vi "Self Execution.vi"(6 "Any Data":variant, 8 "error in (no error)":errorcluster, 9 "Composite Task In":refnum<class "Composite Task.lvclass">, 10 "Message In":refnum<class "Message.lvclass">, 11 "Actor In":refnum<class "System Actor.lvclass">) -> (0 "error out":errorcluster, 1 "Composite Task Out":refnum<class "Composite Task.lvclass">, 2 "Message Out":refnum<class "Message.lvclass">)   [LabVIEW 2019, in "Composite Task.lvclass"]
uses:
  Composite Task.lvclass
  Actor/System Actor/System Actor.lvclass
  Message/Message.lvclass
  Messenger/Messenger/Messenger.lvclass
  Message/Type Def/CMD Type.ctl
  Message/Type Def/General CMD.ctl
  Composite Task.lvclass/Composite Task.ctl
  Message/Message.lvclass/Message.ctl
  Message/Public Data/Write CMD Type.vi
  Message/Public Data/Write General CMD.vi
  Message/Public Data/Write Single Task.vi
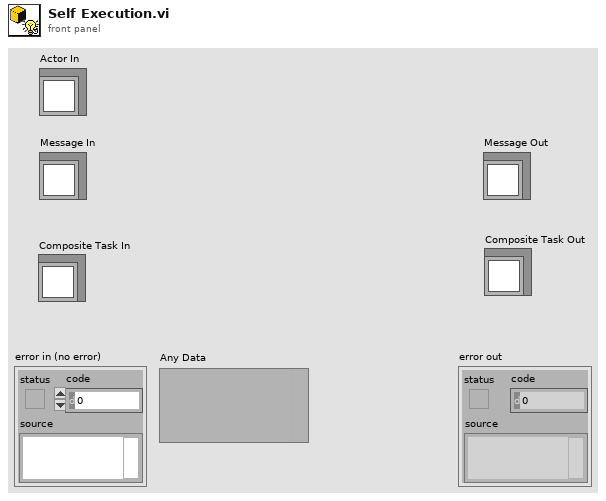
[diagram p1: front panel]
types:
  T1 = typedef "General CMD.ctl" = enum16{"None", "Stop", "Abort", "Running Task", "Running Batch Tasks", "Task Self Running", "Emergency Stop"}
  T2 = typedef "CMD Type.ctl" = enum16{"None", "General CMD", "1st CMD", "2nd CMD", "3rd CMD", "4th CMD", "5th CMD", "6th CMD", "7th CMD"}
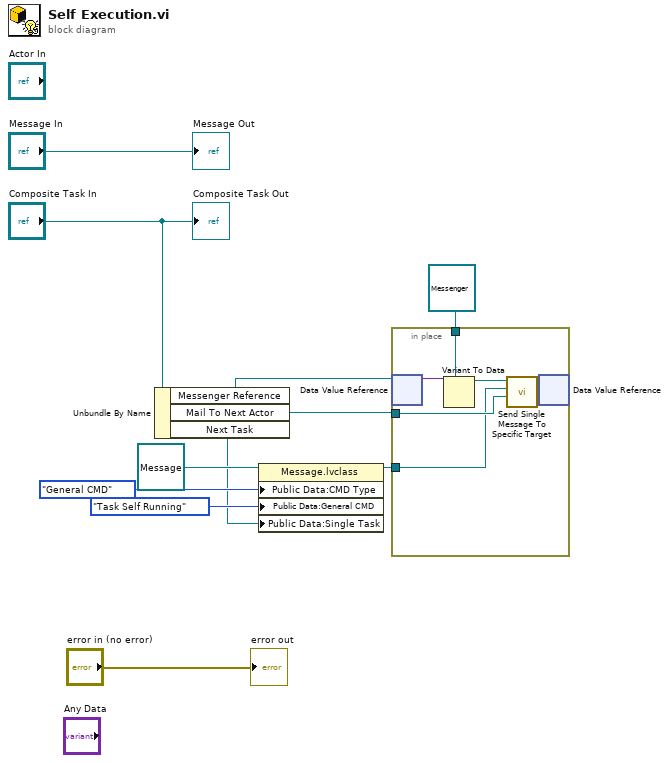
[diagram p0: block diagram]
diagram:
  n1 = Unbundle By Name("Composite Task In") -> ("Messenger Reference"=w7:refnum<data-value>, "Mail To Next Actor"=w8:refnum<class "Mail Strategy.lvclass">, "Next Task"=w2:refnum<class "Task Ancestor.lvclass">)
  n2 = property class="Message.lvclass"(reference=refnum<class "Message.lvclass"> refnum ("Message.lvclass"), "Public Data:CMD Type"=CMD_Type."General CMD" ("CMD Type"), "Public Data:General CMD"=General_CMD."Task Self Running" ("General CMD"), "Public Data:Single Task"=w2) -> (reference out=w1:refnum<class "Message.lvclass">)  [unwired: 1 in, 1 out]
  n3 = in-place {
    in-place-border: w8 -> [w14]
    in-place-border: refnum<class "Messenger.lvclass"> refnum ("Messenger.lvclass") -> [w16]
    in-place-border: w1 -> [w12]
    n4 = in-place-dvr #1(w7) -> (w17:variant)  [unwired: 1 out]
    n5 = Variant To Data(type=w16, Variant=w17) -> (data=w15:refnum<class "Messenger.lvclass">)  [unwired: 1 in, 1 out]
    n6 = call-dynamic "Send Single Message To Specific Target.vi"("Mail Strategy In"=w14, "Message In"=w12, "Messenger in"=w15) -> ("Messenger out"=w13:refnum<class "Messenger.lvclass">)  [unwired: 7 in, 1 out]
    n7 = in-place-dvr #1(w13) -> ()  [unwired: 2 out]
  }
  "error out" <- "error in (no error)"
  "Message Out" <- "Message In"
  "Composite Task Out" <- "Composite Task In"
